vi "LED_Light_Stimulation.vi"() -> ()   [LabVIEW 2009]
uses:
  <vilib>/Utility/file.llb/Read From Spreadsheet File (DBL).vi
panel:
  out "Duration of the Stimulation (s)":i32
  out "Length of the csv file":i32
  out "Light Stimulation DATA (V)":dbl[](graph)
  in  "Set frame size (min=2ms)":u32=33
  in  "Stimulation START":bool
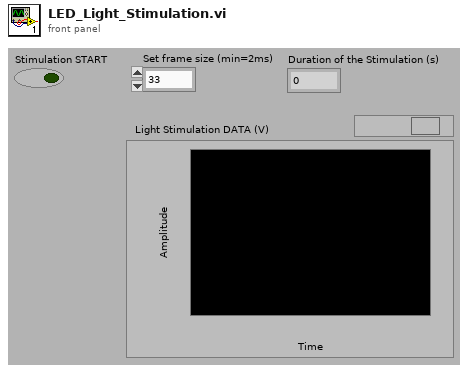
[diagram p1: front panel]
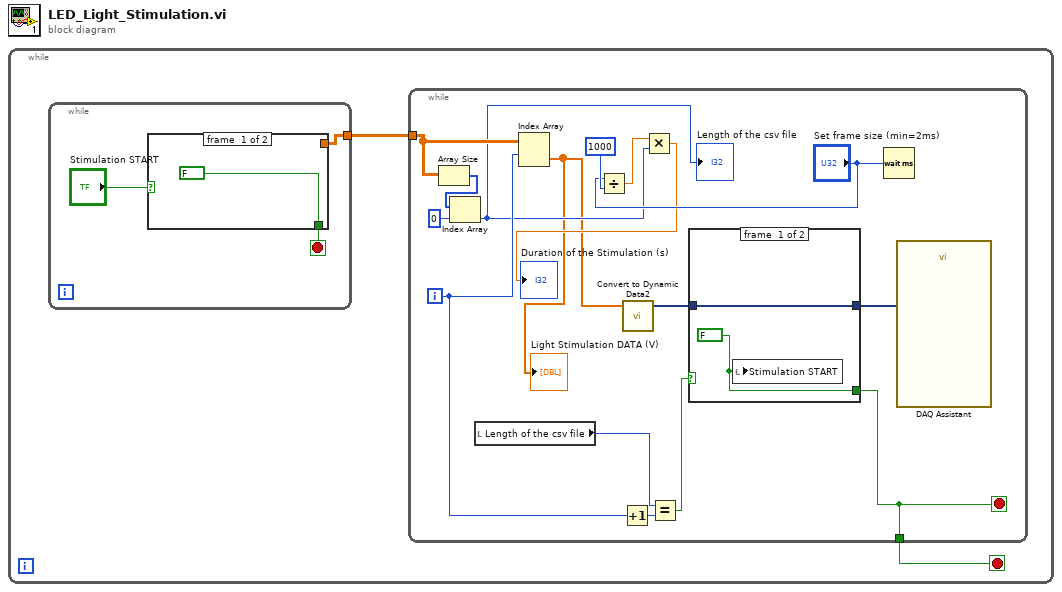
[diagram p0: block diagram]
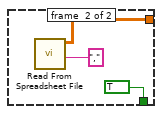
[diagram p2: hidden frame]
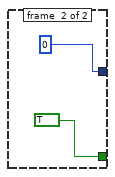
[diagram p3: hidden frame]
diagram:
  n1 = while {
    stop <- w1 stop-if-true
    n2 = while {
      tunnel: [w4] -> w2
      stop <- w3 stop-if-true
      n3 = case shown="False" "Stimulation START" {
        tunnel: [_ w9] -> w4
        tunnel: [FALSE TRUE] -> w3
        frame #0 {
        }
        frame #1 {
          n4 = call-poly <vilib>:"Read From Spreadsheet File.vi"("delimiter (\\t)"="," ("delimiter (\\t)")) -> ("all rows"=w9:dbl[][])  [unwired: 6 in, 4 out]
        }
      }
    }
    n5 = while {
      tunnel: w2 -> [w25]
      tunnel: [w18] -> w1
      i -> [w19]
      stop <- w18 stop-if-true
      n6 = Array Size(array=w25) -> (size(s)=w22:i32[])
      n7 = Index Array(array=w22, index=0) -> (element=w11:i32)
      "Length of the csv file" <- w11
      n8 = local read "Length of the csv file"() -> (w23:i32)
      n9 = Index Array(array=w25, index (row)=w19) -> (element=w10:dbl[])  [unwired: 1 in]
      "Light Stimulation DATA (V)" <- w10
      n10 = Divide(x="Set frame size (min=2ms)", y=1000 ("index")) -> (x/y=w13:dbl)
      n11 = Increment(x=w19) -> (x+1=w20:i32)
      n12 = call "Convert to Dynamic Data2"("Array"=w10) -> ("Dynamic Data Type"=w17:dynamicdata)  [unwired: 3 in]
      n13 = Multiply(x=w13, y=w11) -> (x*y=→"Duration of the Stimulation (s)":dbl)
      n14 = Equal?(x=w23, y=w20) -> (x = y?=w24:bool)
      n15 = case shown="False" w24 {
        tunnel: [w27 TRUE] -> w18
        tunnel: w17 -> [w26 _]
        tunnel: [w26 0] -> w16
        frame #0 {
          w27 = FALSE
          n16 = local write "Stimulation START"(w27) -> ()
        }
        frame #1 {
        }
      }
      n17 = Wait (ms)(milliseconds to wait="Set frame size (min=2ms)") -> ()  [unwired: 1 out]
      n18 = call "DAQ Assistant"("data"=w16) -> ()  [unwired: 17 in, 2 out]
    }
  }
